vi "S2 Step Run For Program.vi"(8 "error in (no error)":errorcluster) -> (0 "error out":errorcluster)   [LabVIEW 2019]
uses:
  LineScan/LineScan.lvclass
  Ctrl/Station Action.ctl
  Ctrl/StationCmdSelect.ctl
  Ctrl/Auto Inspection Station Name2.ctl
  Ctrl/Auto Inspection Data Name.ctl
  Ctrl/MeasureDisplayTab.ctl
  Ctrl/Table Save.ctl
  Ctrl/S2 Station IO.ctl
  Global/Process Global.vi
  LLB/Commonly VI/Main Glb.vi
  LLB/Commonly VI.lvlib
panel:
  out "CurrentCmd 2":string
  out "retry次數 2":string[](array[string])
  out "Retry 2":i32
  in  "Table Control":string[][](table)=[["PCBA BARCODE", ""], ["硬體(Tool初始化)", ""], ["company(Tool初始化)", ""], ["耗電流 uA(電流表)", "T"], ["電池負載電壓", "T"], ["晶片ID(Tool FORMAT)", "F"], ["雷雕ID(TOOl scan、藍芽接收器)", "S"], ["Format(Tool FORMAT)", "F"], ["Programe(Tool Programe)", "P"]]
  out "Numeric":dbl
  out "subarray":string[](array[string])
  out "Program1 receive 2":string
  out "ToolStringOut_P1":string
  out "ToolStringOut_P1_2":string
  out "present":i32
  out "Retry":i32
  out "Act Step":i32
  out "retry次數":string[](array[string])
  out "CurrentCmd":string
  out "Station Out":T1=enum."ImformOut"
  out "LineScan out":refnum<class "LineScan.lvclass">
  in  "LineScan in":refnum<class "LineScan.lvclass">
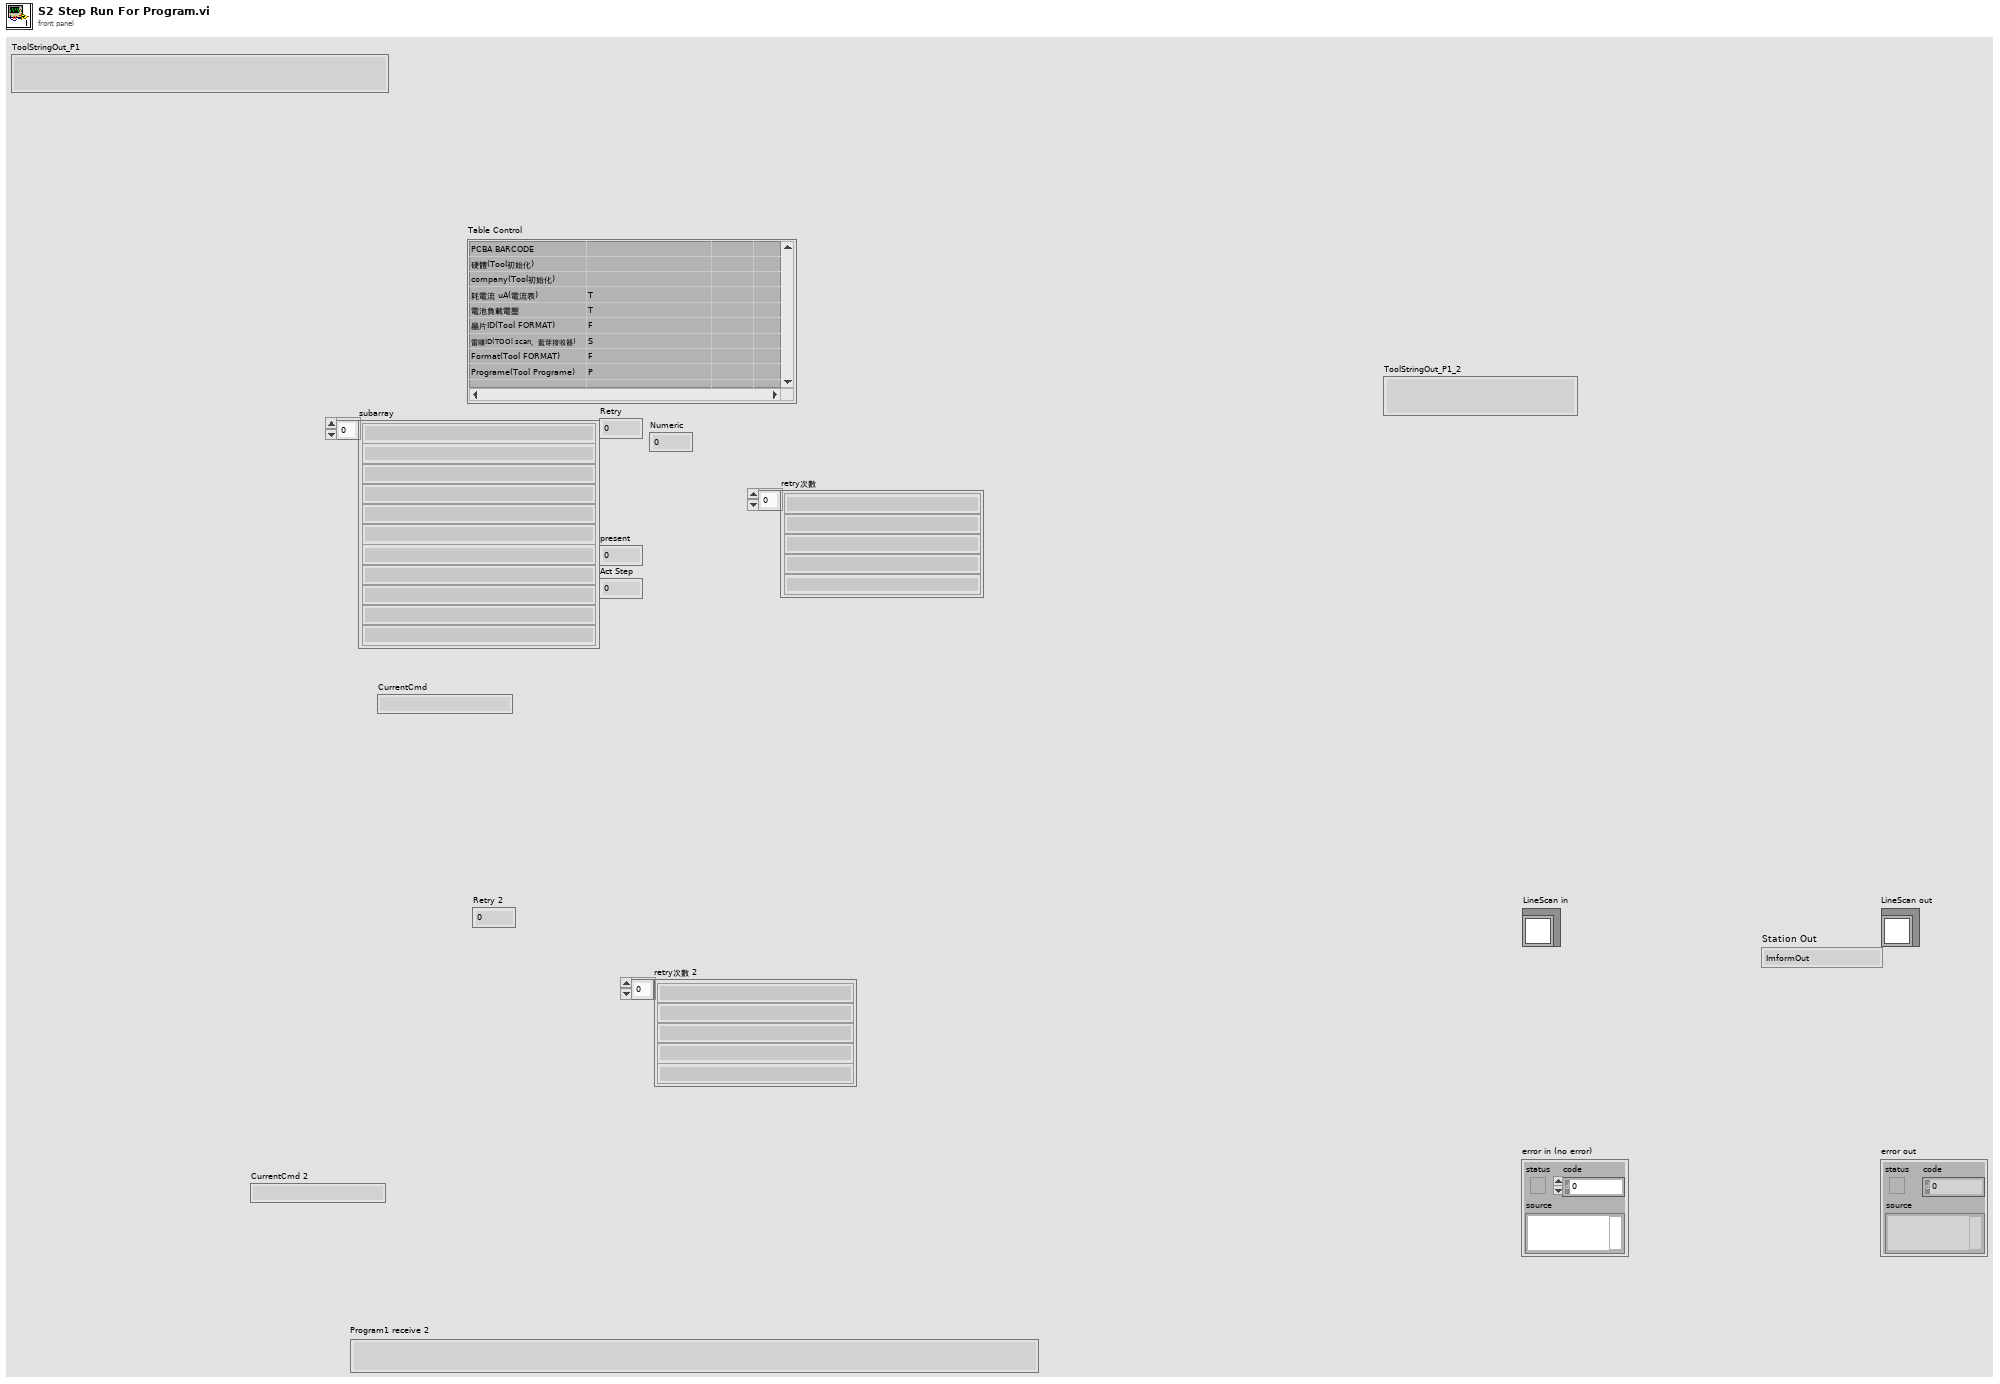
[diagram p1: front panel]
types:
  T1 = typedef "Station Action.ctl" = enum16{"Wait Item In", "Dectect Action", "ImformOut"}
  T2 = typedef "StationCmdSelect.ctl" = enum16{"Action", "Command", "Return", "DTime", "Retry"}
  T3 = typedef "Table Save.ctl" = enum16{"initial", "Add", "Write", "Replace", "Delete", "REad", "RedTable", "Load"}
  T4 = typedef "MeasureDisplayTab.ctl" = enum16{"Tray Barcode", "PCBA BARCODE", "硬體(Tool初始化)", "company(Tool初始化)", "耗電流 uA(電流表)", "電池負載電壓", "晶片ID(Tool FORMAT)", "雷雕ID(TOOl scan、藍芽接收器)", "Format(Tool FORMAT)", "Programe(Tool Programe)", "MAC(藍芽接收器)", "ID(藍芽接收器)", "KPA(藍芽接收器)", "溫度(藍芽接收器)", "SENSOR電池電壓(藍芽接收器)", "RSSI(藍芽接收器)", "SensorType_315(FSK scan)", "FSKsnVol_315(FSK scan)", "FSKscanl_315(FSK scan)", "P_315(FSK scan)", "T_315(FSK scan)", "SensorType_433(ASK scan)", "ASKsnVol_433(ASK scan)", "ASKscan_433(ASK scan)", "P_433(ASK scan)", "T_433(ASK scan)", "測高Data"}
  T5 = typedef "Auto Inspection Data Name.ctl" = enum16{"LocalRun", "ItemSN(TimeCode)", "CurrentAction", "Error", "Data", "OKNG", "電壓值", "電壓值判斷", "電流值", "電流值判斷", "Laser1 Data", "Laser2 Data", "Laser OKNG", "StationNO"}
  T6 = typedef "Auto Inspection Station Name2.ctl" = enum16{"S1Barcode", "S2Measure", "S3Measure", "S4Measure", "S5Measure", "S11_LaserCheck", "S8_Vision AI"}
  T7 = typedef "S2 Station IO.ctl" = enum16{"S2站PC動作中_20", "電流量測完成產品OK_21", "電流量測完成產品NG_22", "S2站Format 執行_23", "S2 Format OK_24", "S2 Format NG_25", "S2站燒入執行_26", "S2站燒入OK_27", "S2站燒入NG_28", "S2站動作完成_29", "S3 PC動作中_30", "S3 Format 此站執行_31", "S3 Format OK_32", "S3 Format NG_33", "S3 燒入程式 此站執行_34", "S3 燒入程式 OK_35", "S3 燒入程式 NG_36", "S3 備用_37", "S3 備用_38", "S3 動作完成_39", "S4 PC動作中_40", "S4 量測完成 產品正常_41", "S4 量測完成 產品NG_42", "S4 Format 此站執行_43", "S4 Format OK_44", "S4 Format NG_45", "S4 燒入 此站不執行_46", "S4 燒入程式 OK_47", "S4 燒入程式 NG_48", "S4 藍芽Scan OK_49", "S4 藍芽Scan NG_50", "S4 動作完成_51", "給PLC要量電流訊號", "給PLC要量電壓訊號"}
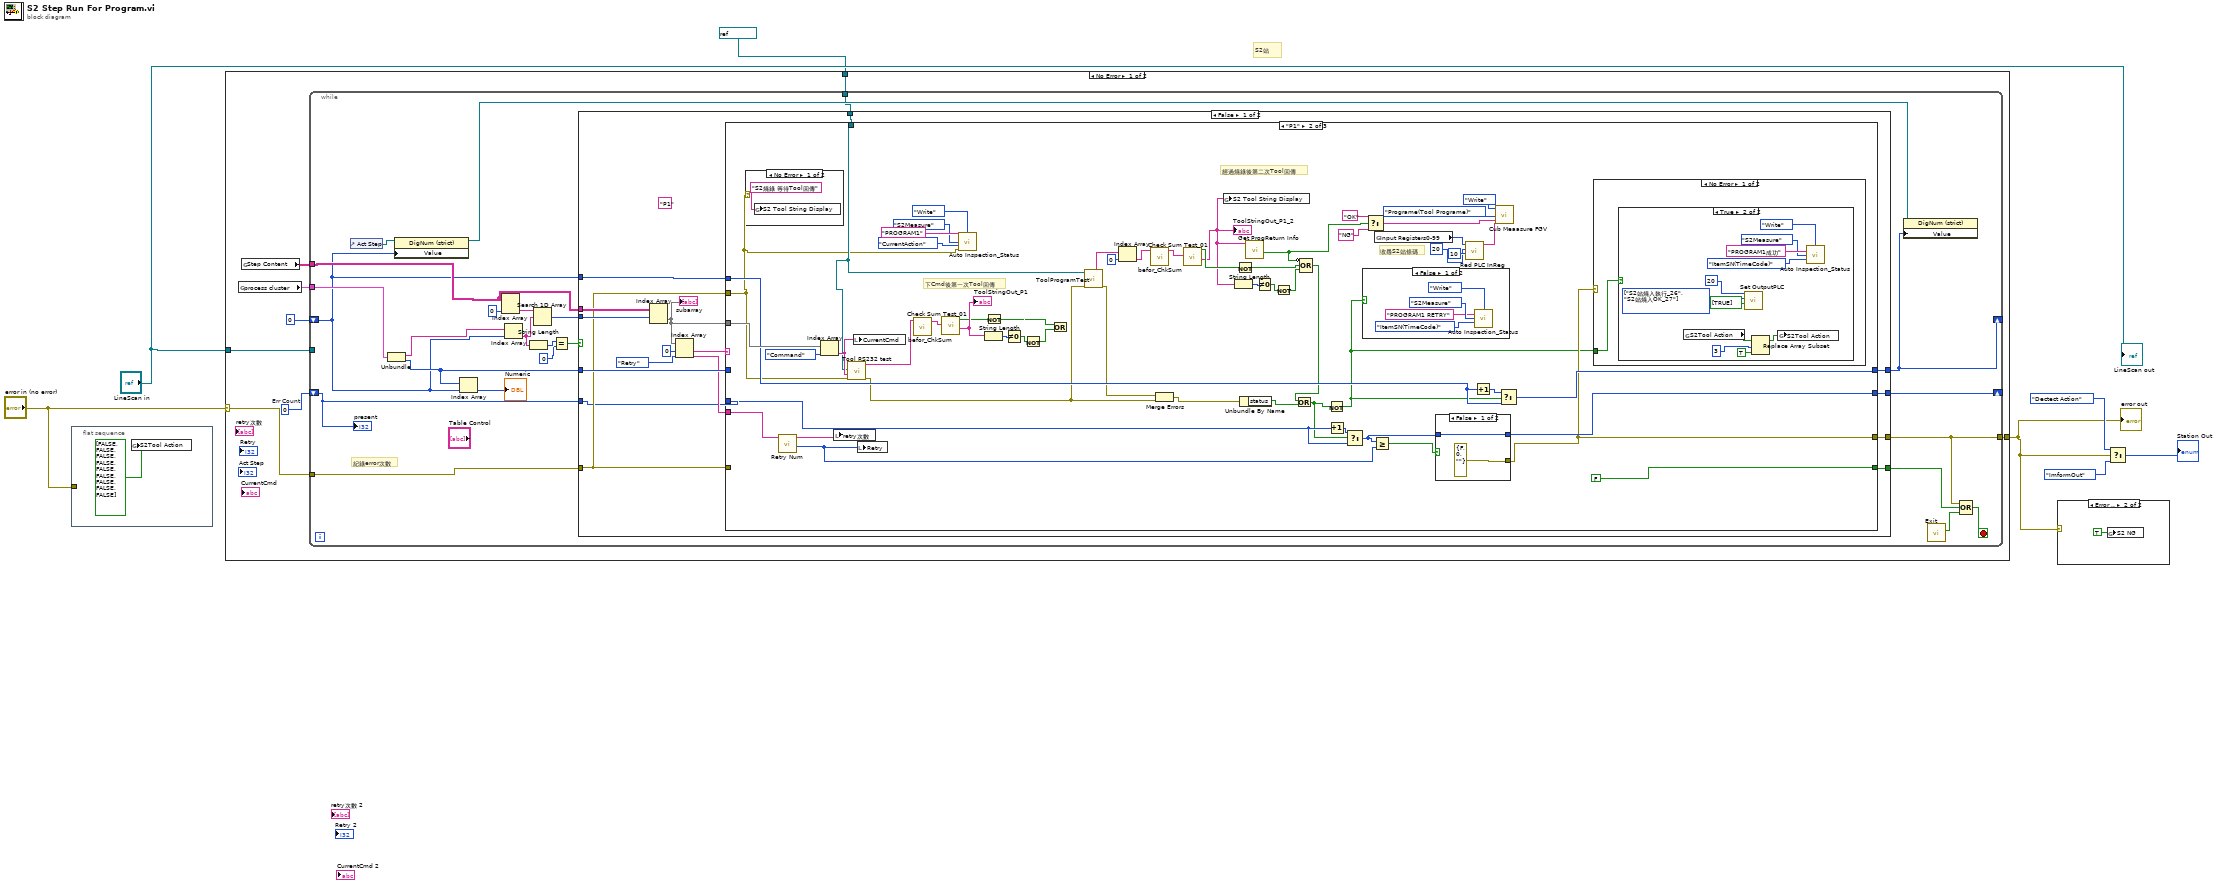
[diagram p0: block diagram]
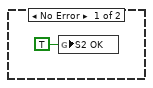
[diagram p2: hidden frame]
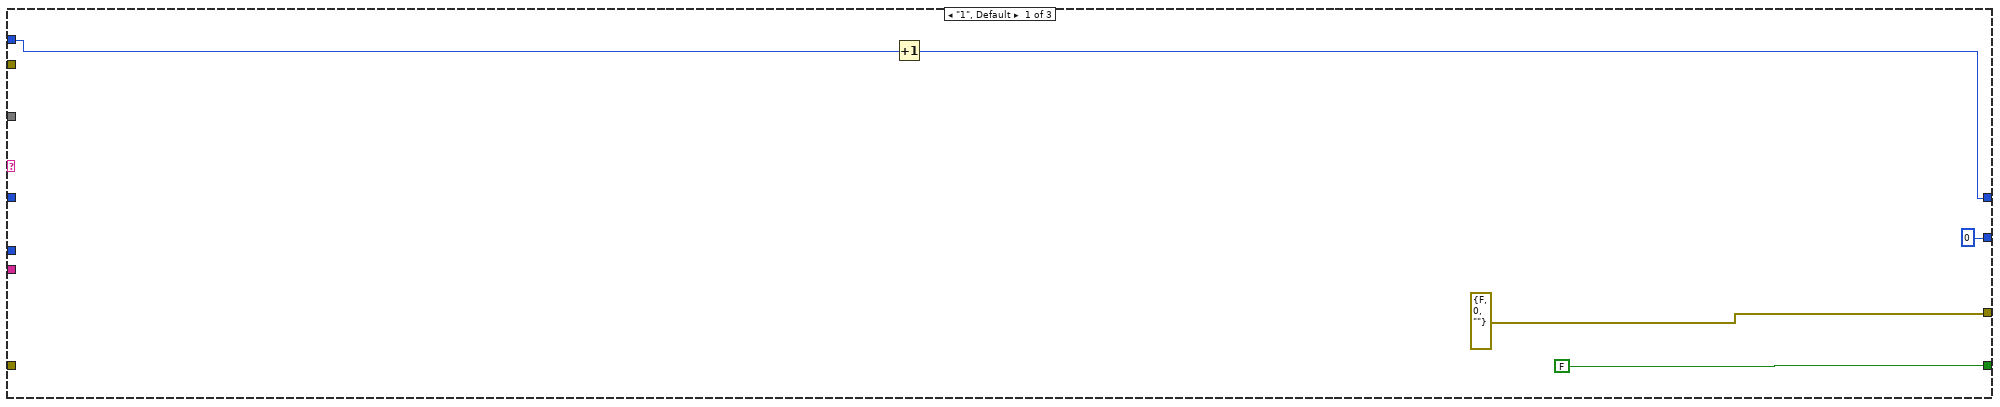
[diagram p3: hidden frame]
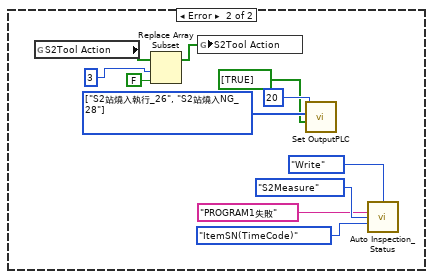
[diagram p7: hidden frame]
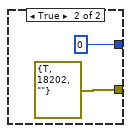
[diagram p8: hidden frame]
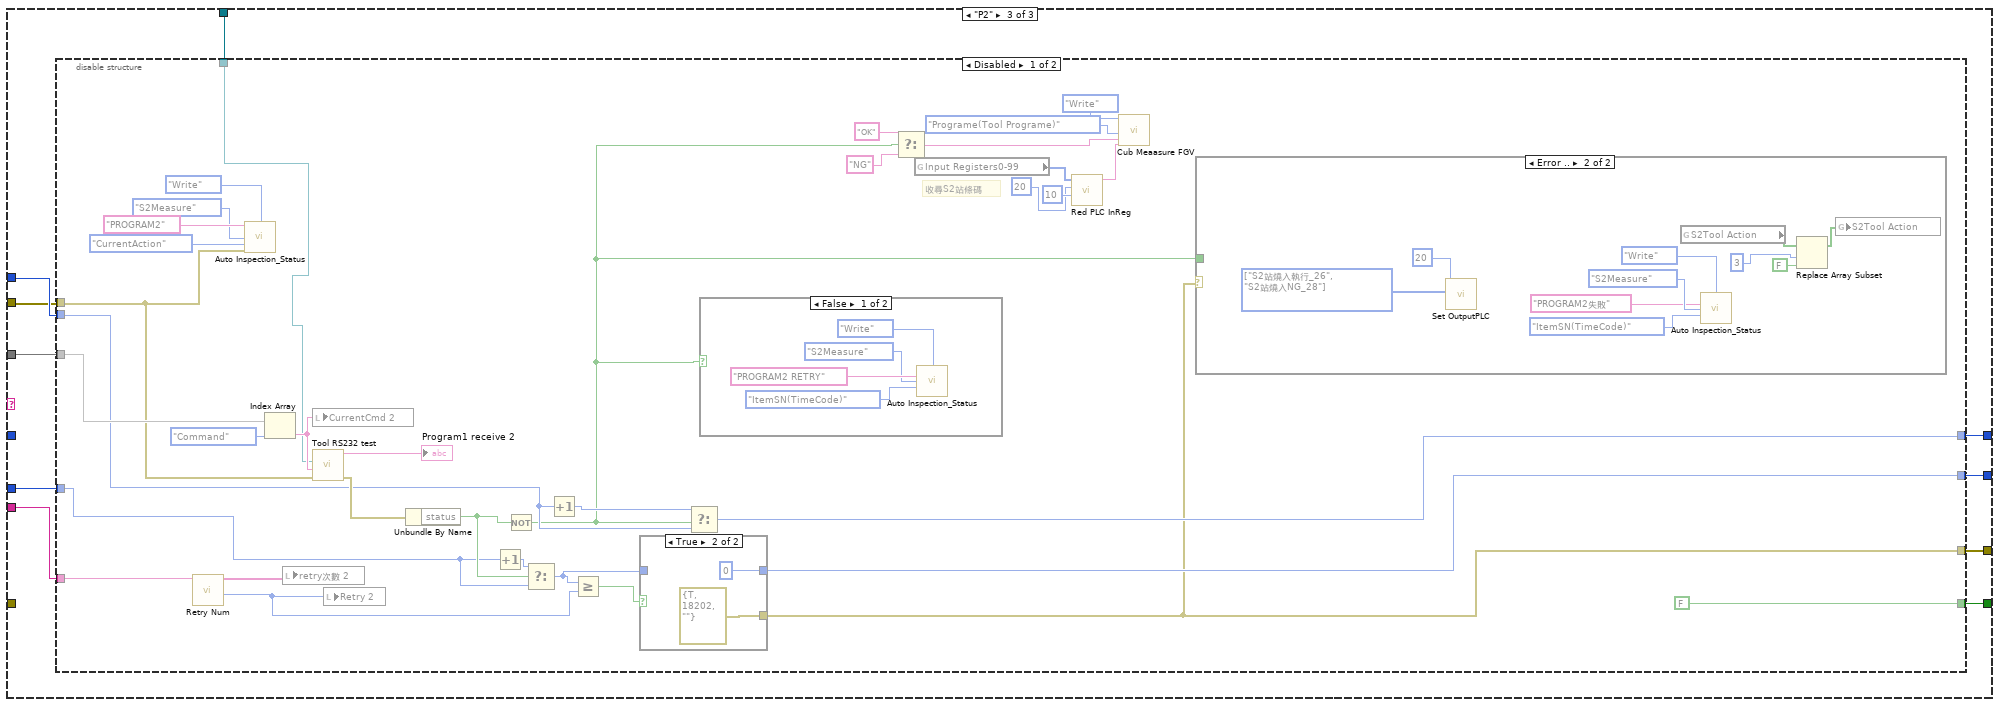
[diagram p9: hidden frame]
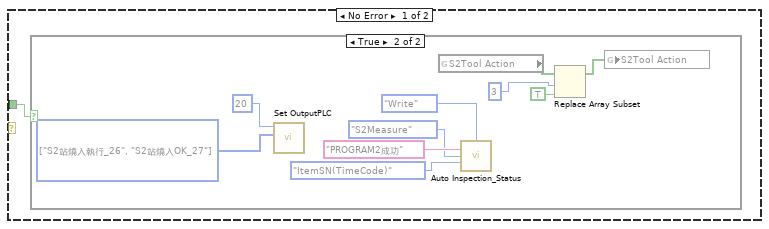
[diagram p11: hidden frame]
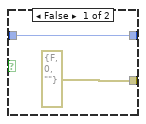
[diagram p13: hidden frame]
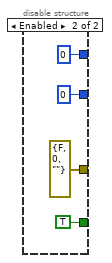
[diagram p14: hidden frame]
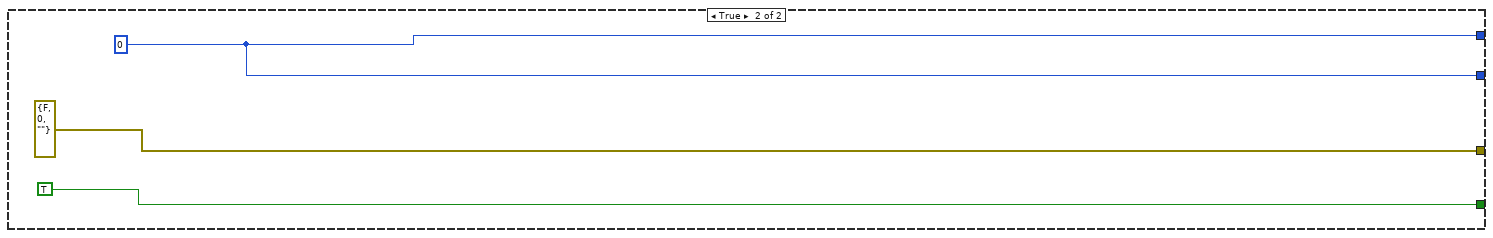
[diagram p15: hidden frame]
diagram:
  # "S2站"
  n1 = flat-sequence {
    tunnel: "error in (no error)" -> [_]
    frame #0 {
      n2 = global write "Process Global.vi" "S2Tool Action"(bool[] [FALSE, FALSE, FALSE, FALSE, FALSE, FALSE, FALSE, FALSE, FALSE] ("S2Tool Action")) -> ()
    }
  }
  n3 = case shown="No Error" "error in (no error)" {
    selector: "error in (no error)" -> [w10 w232]
    tunnel: [w16 w232] -> w2
    tunnel: "LineScan in" -> [w15 _]
    tunnel: refnum<visa-resource-name> "COM1" ("VISA resource name") -> [w9 _]
    frame No Error {
      w11 = 0  # Err Count
      n4 = global read "Process Global.vi" "process cluster"() -> (w13:cluster{string[], i32[]})
      n5 = global read "Process Global.vi" "Step Content"() -> (w14:string[][])
      n6 = while {
        tunnel: [w26] -> w16
        shift-right: [w22] -> _
        shift-left: 0 -> [w23]
        tunnel: w15 -> [_]
        shift-right: [w19] -> _
        shift-left: w11 -> [w25]
        tunnel: w14 -> [w37]
        tunnel: w13 -> [w36]
        tunnel: w10 -> [w20]
        tunnel: w9 -> [w18]
        stop <- w38 stop-if-true
        # "紀錄error次數"
        n7 = control-ref of="Act Step"() -> (w24:refnum<vi>)
        n8 = Unbundle(w36) -> (w39:string[], w40:i32[])
        n9 = property class="DigNum (strict)"(reference=w24, "Value"=w23) -> (reference out=w21:refnum<vi>)  [unwired: 1 in, 1 out]
        n10 = Index Array(array=w40, index=w23) -> (element=→"Numeric":i32)
        n11 = Index Array(array=w37, index (col)=0 ("disabled index (col)")) -> (element=w34:string[])  [unwired: 1 in]
        n12 = Index Array(array=w39, index=w23) -> (element=w30:string)
        n13 = String Length(string=w30) -> (length=w31:i32)
        n14 = Search 1D Array(1D array=w34, element=w30) -> (index of element=w33:i32)  [unwired: 1 in]
        n15 = Equal?(x=w31, y=0) -> (x = y?=w28:bool)
        n16 = case shown="False" w28 {
          tunnel: w40 -> [w56 _]
          tunnel: w37 -> [w55 _]
          tunnel: w33 -> [w54 _]
          tunnel: [w46 TRUE] -> w27
          tunnel: [w48 errorcluster {"status"=FALSE, "code"=0, "source"=""} ("error constant")] -> w26
          tunnel: w23 -> [w50 _]
          tunnel: [w49 w229] -> w22
          tunnel: w25 -> [w44 _]
          tunnel: w20 -> [w45 _]
          tunnel: [w43 w229] -> w19
          tunnel: w18 -> [w42 _]
          frame False {
            (unwired) "P1"
            n17 = Index Array(array=w55, index (row)=w54) -> (element=w51:string[])  [unwired: 1 in]
            "subarray" <- w51
            n18 = Index Array(array=w51, index #1=0 ("index"), index #2=StationCmdSelect."Retry") -> (element #1=w41:string, element #2=w52:string)
            n19 = case shown="\"P1\"" w41 {
              tunnel: w56 -> [_ _ _]
              tunnel: w52 -> [_ w108 w156]
              tunnel: w51 -> [_ w110 w159]
              tunnel: w50 -> [w61 w109 w158]
              tunnel: [w60 w107 w155] -> w49
              tunnel: [errorcluster {"status"=FALSE, "code"=0, "source"=""} ("error constant") w68 w152] -> w48
              tunnel: [FALSE FALSE w153] -> w46
              tunnel: w45 -> [_ _ _]
              tunnel: w45 -> [_ w66 w151]
              tunnel: w44 -> [_ w91 w157]
              tunnel: [0 ("Err Count") w92 w154] -> w43
              tunnel: w42 -> [_ w82 w160]
              frame "1", Default {
                n20 = Increment(x=w61) -> (x+1=w60:i32)
              }
              frame "P1" {
                # "經過燒錄後第二次Tool回傳"
                # "下Cmd後第一次Tool回傳"
                # "收尋S2站條碼"
                n21 = case shown="No Error" w66 {
                  frame No Error {
                    n22 = global write "Process Global.vi" "S2 Tool String Display"("S2燒錄 等待Tool回傳" ("S2 Tool String Display")) -> ()
                  }
                  frame Error {
                  }
                }
                n23 = call "Retry Num.vi"("String"=w108) -> ("Numeric"=w116:i32, "retry次數"=w113:string[])  [unwired: 9 in]
                n24 = Index Array(array=w110, index=StationCmdSelect."Command") -> (element=w112:string)
                n25 = local write "retry次數"(w113) -> ()
                n26 = call "Tool RS232 test.vi"("error in (no error)"=w66, "Cmd In"=w112, "VISA resource name"=w82) -> ("error out"=w63:errorcluster, "receive string"=w83:string)  [unwired: 7 in]
                n27 = local write "CurrentCmd"(w112) -> ()
                n28 = local write "Retry"(w116) -> ()
                n29 = call "befor_ChkSum.vi"("ToolString Input"=w83) -> ("Array"=w84:string[])  [unwired: 9 in, 1 out]
                n30 = call "Check Sum Test_01.vi"("Array"=w84) -> ("ToolStringOut_01"=w87:string, "x = y?"=w85:bool)  [unwired: 8 in, 1 out]
                "ToolStringOut_P1" <- w87
                n31 = call "Auto Inspection_Status.vi"("Action"=enum16{"Initial", "Write", "Read"}."Write", "DataIn"="PROGRAM1", "Station"=Auto_Inspection_Station_Name2."S2Measure", "Data"=Auto_Inspection_Data_Name."CurrentAction", "error in"=w66) -> ()  [unwired: 8 in, 3 out]
                n32 = String Length(string=w87) -> (length=w89:i32)
                n33 = Not(x=w85) -> (.not. x?=w86:bool)
                n34 = Not Equal To 0?(x=w89) -> (x != 0?=w90:bool)
                n35 = Not(x=w90) -> (.not. x?=w88:bool)
                n36 = Or(x=w86, y=w88) -> ()  [unwired: 1 out]
                n37 = call "ToolProgramTest.vi"("error in (no error)"=w63, "VISA resource name"=w82) -> ("error out"=w64:errorcluster, "Array"=w73:string[])  [unwired: 4 in, 4 out]
                n38 = Index Array(array=w73, index=0) -> (element=w80:string)
                n39 = call "befor_ChkSum.vi"("ToolString Input"=w80) -> ("Array"=w79:string[])  [unwired: 9 in, 1 out]
                n40 = Merge Errors(w64, w63) -> (w62:errorcluster)
                n41 = call "Check Sum Test_01.vi"("Array"=w79) -> ("ToolStringOut_01"=w67:string, "x = y?"=w76:bool)  [unwired: 8 in, 1 out]
                "ToolStringOut_P1_2" <- w67
                n42 = global write "Process Global.vi" "S2 Tool String Display"(w67) -> ()
                n43 = String Length(string=w67) -> (length=w77:i32)
                n44 = Not(x=w76) -> (.not. x?=w75:bool)
                n45 = Unbundle By Name(w62) -> ("status"=w71:bool)
                n46 = call "Get ProgReturn Info.vi"("String"=w67) -> ("Chk OK or Fail"=w72:bool)  [unwired: 8 in, 2 out]
                n47 = Not Equal To 0?(x=w77) -> (x != 0?=w78:bool)
                n48 = Not(x=w78) -> (.not. x?=w74:bool)
                n49 = Compound Arithmetic op=OR(invert w72, w75, w74) -> (w70:bool)
                n50 = Or(x=w70, y=w71) -> (x .or. y?=w69:bool)
                n51 = Not(x=w69) -> (.not. x?=w65:bool)
                n52 = Increment(x=w91) -> (x+1=w117:i32)
                n53 = Select(t=w117, s=w69, f=w91) -> (s? t:f=w114:i32)
                n54 = case shown="False" w65 {
                  frame False {
                    n55 = call "Auto Inspection_Status.vi"("Action"=enum16{"Initial", "Write", "Read"}."Write", "DataIn"="PROGRAM1 RETRY", "Station"=Auto_Inspection_Station_Name2."S2Measure", "Data"=Auto_Inspection_Data_Name."ItemSN(TimeCode)") -> ()  [unwired: 9 in, 3 out]
                  }
                  frame True {
                  }
                }
                n56 = Select(t="OK" ("DataIn"), s=w72, f="NG" ("DataIn")) -> (s? t:f=w101:string)
                n57 = Greater Or Equal?(x=w114, y=w116) -> (x >= y?=w115:bool)
                n58 = global read "Main Glb.vi" "Input Registers0-99"() -> (w94:u16[])
                n59 = case shown="False" w115 {
                  tunnel: [errorcluster {"status"=FALSE, "code"=0, "source"=""} ("error constant") errorcluster {"status"=TRUE, "code"=18202, "source"=""} ("error constant")] -> w68
                  tunnel: w114 -> [w147 _]
                  tunnel: [w147 0] -> w92
                  frame False {
                  }
                  frame True {
                  }
                }
                n60 = call "Red PLC InReg.vi"("length"=10, "index"=20, "Input Registers Arr"=w94) -> ("Rad In Reg"=w95:string)  [unwired: 7 in, 1 out]
                n61 = Increment(x=w109) -> (x+1=w118:i32)
                n62 = call "Cub Meaasure FGV.vi"("Action"=Table_Save."Write" ("Enum"), "Save Index"=MeasureDisplayTab."Programe(Tool Programe)", "DataIn"=w101, "SN"=w95) -> ()  [unwired: 8 in, 8 out]
                n63 = Select(t=w118, s=w65, f=w109) -> (s? t:f=w107:i32)
                n64 = case shown="No Error" w68 {
                  tunnel: w65 -> [w124 _]
                  frame No Error {
                    n65 = case shown="True" w124 {
                      frame False {
                      }
                      frame True {
                        w134 = T7[] [enum."S2站燒入執行_26", enum."S2站燒入OK_27"] items=["S2站PC動作中_20", "電流量測完成產品OK_21", "電流量測完成產品NG_22", "S2站Format 執行_23", "S2 Format OK_24", "S2 Format NG_25", "S2站燒入執行_26", "S2站燒入OK_27", "S2站燒入NG_28", "S2站動作完成_29", "S3 PC動作中_30", "S3 Format 此站執行_31", "S3 Format OK_32", "S3 Format NG_33", "S3 燒入程式 此站執行_34", "S3 燒入程式 OK_35", "S3 燒入程式 NG_36", "S3 備用_37", "S3 備用_38", "S3 動作完成_39", "S4 PC動作中_40", "S4 量測完成 產品正常_41", "S4 量測完成 產品NG_42", "S4 Format 此站執行_43", "S4 Format OK_44", "S4 Format NG_45", "S4 燒入 此站不執行_46", "S4 燒入程式 OK_47", "S4 燒入程式 NG_48", "S4 藍芽Scan OK_49", "S4 藍芽Scan NG_50", "S4 動作完成_51", "給PLC要量電流訊號", "給PLC要量電壓訊號"]
                        n66 = global read "Process Global.vi" "S2Tool Action"() -> (w129:bool[])
                        n67 = call "Set OutputPLC.vi"("Address In"=20, "Array 2"=w134, "Sat Coils"=bool[] [TRUE]) -> ()  [unwired: 7 in, 1 out]
                        n68 = Replace Array Subset(array=w129, new element=TRUE ("new element/subarray"), index=3) -> (w126:bool[])
                        n69 = global write "Process Global.vi" "S2Tool Action"(w126) -> ()
                        n70 = call "Auto Inspection_Status.vi"("Action"=enum16{"Initial", "Write", "Read"}."Write", "DataIn"="PROGRAM1成功", "Station"=Auto_Inspection_Station_Name2."S2Measure", "Data"=Auto_Inspection_Data_Name."ItemSN(TimeCode)") -> ()  [unwired: 9 in, 3 out]
                      }
                    }
                  }
                  frame Error {
                    w146 = T7[] [enum."S2站燒入執行_26", enum."S2站燒入NG_28"] items=["S2站PC動作中_20", "電流量測完成產品OK_21", "電流量測完成產品NG_22", "S2站Format 執行_23", "S2 Format OK_24", "S2 Format NG_25", "S2站燒入執行_26", "S2站燒入OK_27", "S2站燒入NG_28", "S2站動作完成_29", "S3 PC動作中_30", "S3 Format 此站執行_31", "S3 Format OK_32", "S3 Format NG_33", "S3 燒入程式 此站執行_34", "S3 燒入程式 OK_35", "S3 燒入程式 NG_36", "S3 備用_37", "S3 備用_38", "S3 動作完成_39", "S4 PC動作中_40", "S4 量測完成 產品正常_41", "S4 量測完成 產品NG_42", "S4 Format 此站執行_43", "S4 Format OK_44", "S4 Format NG_45", "S4 燒入 此站不執行_46", "S4 燒入程式 OK_47", "S4 燒入程式 NG_48", "S4 藍芽Scan OK_49", "S4 藍芽Scan NG_50", "S4 動作完成_51", "給PLC要量電流訊號", "給PLC要量電壓訊號"]
                    n71 = global read "Process Global.vi" "S2Tool Action"() -> (w140:bool[])
                    n72 = Replace Array Subset(array=w140, new element=FALSE ("new element/subarray"), index=3) -> (w137:bool[])
                    n73 = global write "Process Global.vi" "S2Tool Action"(w137) -> ()
                    n74 = call "Set OutputPLC.vi"("Address In"=20, "Array 2"=w146, "Sat Coils"=bool[] [TRUE]) -> ()  [unwired: 7 in, 1 out]
                    n75 = call "Auto Inspection_Status.vi"("Action"=enum16{"Initial", "Write", "Read"}."Write", "DataIn"="PROGRAM1失敗", "Station"=Auto_Inspection_Station_Name2."S2Measure", "Data"=Auto_Inspection_Data_Name."ItemSN(TimeCode)") -> ()  [unwired: 9 in, 3 out]
                  }
                }
              }
              frame "P2" {
                n76 = disable-structure shown="Disabled" {
                  disable-tunnel: w160 -> [w171 _]
                  disable-tunnel: w159 -> [w170 _]
                  disable-tunnel: w158 -> [w169 _]
                  disable-tunnel: w157 -> [w168 _]
                  disable-tunnel: w156 -> [w167 _]
                  disable-tunnel: [w166 0] -> w155
                  disable-tunnel: [w165 0 ("Err Count")] -> w154
                  disable-tunnel: [FALSE TRUE] -> w153
                  disable-tunnel: [w163 errorcluster {"status"=FALSE, "code"=0, "source"=""} ("error constant")] -> w152
                  disable-tunnel: w151 -> [w162 _]
                  frame Disabled {
                    # "收尋S2站條碼"
                    n77 = call "Retry Num.vi"("String"=w167) -> ("Numeric"=w188:i32, "retry次數"=w191:string[])  [unwired: 9 in]
                    n78 = call "Auto Inspection_Status.vi"("Action"=enum16{"Initial", "Write", "Read"}."Write", "DataIn"="PROGRAM2", "Station"=Auto_Inspection_Station_Name2."S2Measure", "Data"=Auto_Inspection_Data_Name."CurrentAction", "error in"=w162) -> ()  [unwired: 8 in, 3 out]
                    n79 = Index Array(array=w170, index=StationCmdSelect."Command") -> (element=w192:string)
                    n80 = local write "retry次數 2"(w191) -> ()
                    n81 = local write "CurrentCmd 2"(w192) -> ()
                    n82 = call "Tool RS232 test.vi"("error in (no error)"=w162, "Cmd In"=w192, "VISA resource name"=w171) -> ("error out"=w184:errorcluster, "receive string"=→"Program1 receive 2":string)  [unwired: 7 in]
                    n83 = local write "Retry 2"(w188) -> ()
                    n84 = Unbundle By Name(w184) -> ("status"=w186:bool)
                    n85 = Increment(x=w168) -> (x+1=w187:i32)
                    n86 = Not(x=w186) -> (.not. x?=w161:bool)
                    n87 = Select(t=w187, s=w186, f=w168) -> (s? t:f=w190:i32)
                    n88 = Increment(x=w169) -> (x+1=w185:i32)
                    n89 = Greater Or Equal?(x=w190, y=w188) -> (x >= y?=w189:bool)
                    n90 = case shown="True" w189 {
                      tunnel: [errorcluster {"status"=FALSE, "code"=0, "source"=""} ("error constant") errorcluster {"status"=TRUE, "code"=18202, "source"=""} ("error constant")] -> w163
                      tunnel: w190 -> [w221 _]
                      tunnel: [w221 0] -> w165
                      frame False {
                      }
                      frame True {
                      }
                    }
                    n91 = Select(t=w185, s=w161, f=w169) -> (s? t:f=w166:i32)
                    n92 = case shown="False" w161 {
                      frame False {
                        n93 = call "Auto Inspection_Status.vi"("Action"=enum16{"Initial", "Write", "Read"}."Write", "DataIn"="PROGRAM2 RETRY", "Station"=Auto_Inspection_Station_Name2."S2Measure", "Data"=Auto_Inspection_Data_Name."ItemSN(TimeCode)") -> ()  [unwired: 9 in, 3 out]
                      }
                      frame True {
                      }
                    }
                    n94 = Select(t="OK" ("DataIn"), s=w161, f="NG" ("DataIn")) -> (s? t:f=w193:string)
                    n95 = global read "Main Glb.vi" "Input Registers0-99"() -> (w195:u16[])
                    n96 = call "Red PLC InReg.vi"("length"=10, "index"=20, "Input Registers Arr"=w195) -> ("Rad In Reg"=w194:string)  [unwired: 7 in, 1 out]
                    n97 = call "Cub Meaasure FGV.vi"("Action"=Table_Save."Write" ("Enum"), "Save Index"=MeasureDisplayTab."Programe(Tool Programe)", "DataIn"=w193, "SN"=w194) -> ()  [unwired: 8 in, 8 out]
                    n98 = case shown="Error .." w163 {
                      tunnel: w161 -> [w200 _]
                      frame No Error {
                        n99 = case shown="True" w200 {
                          frame False {
                          }
                          frame True {
                            w209 = T7[] [enum."S2站燒入執行_26", enum."S2站燒入OK_27"] items=["S2站PC動作中_20", "電流量測完成產品OK_21", "電流量測完成產品NG_22", "S2站Format 執行_23", "S2 Format OK_24", "S2 Format NG_25", "S2站燒入執行_26", "S2站燒入OK_27", "S2站燒入NG_28", "S2站動作完成_29", "S3 PC動作中_30", "S3 Format 此站執行_31", "S3 Format OK_32", "S3 Format NG_33", "S3 燒入程式 此站執行_34", "S3 燒入程式 OK_35", "S3 燒入程式 NG_36", "S3 備用_37", "S3 備用_38", "S3 動作完成_39", "S4 PC動作中_40", "S4 量測完成 產品正常_41", "S4 量測完成 產品NG_42", "S4 Format 此站執行_43", "S4 Format OK_44", "S4 Format NG_45", "S4 燒入 此站不執行_46", "S4 燒入程式 OK_47", "S4 燒入程式 NG_48", "S4 藍芽Scan OK_49", "S4 藍芽Scan NG_50", "S4 動作完成_51", "給PLC要量電流訊號", "給PLC要量電壓訊號"]
                            n100 = call "Set OutputPLC.vi"("Address In"=20, "Array 2"=w209) -> ()  [unwired: 8 in, 1 out]
                            n101 = global read "Process Global.vi" "S2Tool Action"() -> (w204:bool[])
                            n102 = call "Auto Inspection_Status.vi"("Action"=enum16{"Initial", "Write", "Read"}."Write", "DataIn"="PROGRAM2成功", "Station"=Auto_Inspection_Station_Name2."S2Measure", "Data"=Auto_Inspection_Data_Name."ItemSN(TimeCode)") -> ()  [unwired: 9 in, 3 out]
                            n103 = Replace Array Subset(array=w204, new element=TRUE ("new element/subarray"), index=3) -> (w201:bool[])
                            n104 = global write "Process Global.vi" "S2Tool Action"(w201) -> ()
                          }
                        }
                      }
                      frame Error {
                        w220 = T7[] [enum."S2站燒入執行_26", enum."S2站燒入NG_28"] items=["S2站PC動作中_20", "電流量測完成產品OK_21", "電流量測完成產品NG_22", "S2站Format 執行_23", "S2 Format OK_24", "S2 Format NG_25", "S2站燒入執行_26", "S2站燒入OK_27", "S2站燒入NG_28", "S2站動作完成_29", "S3 PC動作中_30", "S3 Format 此站執行_31", "S3 Format OK_32", "S3 Format NG_33", "S3 燒入程式 此站執行_34", "S3 燒入程式 OK_35", "S3 燒入程式 NG_36", "S3 備用_37", "S3 備用_38", "S3 動作完成_39", "S4 PC動作中_40", "S4 量測完成 產品正常_41", "S4 量測完成 產品NG_42", "S4 Format 此站執行_43", "S4 Format OK_44", "S4 Format NG_45", "S4 燒入 此站不執行_46", "S4 燒入程式 OK_47", "S4 燒入程式 NG_48", "S4 藍芽Scan OK_49", "S4 藍芽Scan NG_50", "S4 動作完成_51", "給PLC要量電流訊號", "給PLC要量電壓訊號"]
                        n105 = call "Set OutputPLC.vi"("Address In"=20, "Array 2"=w220) -> ()  [unwired: 8 in, 1 out]
                        n106 = global read "Process Global.vi" "S2Tool Action"() -> (w214:bool[])
                        n107 = call "Auto Inspection_Status.vi"("Action"=enum16{"Initial", "Write", "Read"}."Write", "DataIn"="PROGRAM2失敗", "Station"=Auto_Inspection_Station_Name2."S2Measure", "Data"=Auto_Inspection_Data_Name."ItemSN(TimeCode)") -> ()  [unwired: 9 in, 3 out]
                        n108 = Replace Array Subset(array=w214, new element=FALSE ("new element/subarray"), index=3) -> (w211:bool[])
                        n109 = global write "Process Global.vi" "S2Tool Action"(w211) -> ()
                      }
                    }
                  }
                  frame Enabled {
                  }
                }
              }
            }
          }
          frame True {
            w229 = 0
          }
        }
        n110 = property class="DigNum (strict)"(reference=w21, "Value"=w22) -> ()  [unwired: 1 in, 2 out]
        n111 = call "Exit.vi"() -> ("ExitOut"=w17:bool)  [unwired: 11 in]
        n112 = Compound Arithmetic op=OR(w26, w27, w17) -> (w38:bool)
        "present" <- w25
      }
    }
    frame Error {
    }
  }
  "error out" <- w2
  n113 = case shown="Error .." w2 {
    frame No Error {
      n114 = global write "Process Global.vi" "S2 OK"(TRUE ("S2 OK")) -> ()
    }
    frame Error {
      n115 = global write "Process Global.vi" "S2 NG"(TRUE ("S2 NG")) -> ()
    }
  }
  n116 = Select(t=Station_Action."Dectect Action" ("Station Out"), s=w2, f=Station_Action."ImformOut" ("Station Out")) -> (s? t:f=→"Station Out":T1)
  "LineScan out" <- "LineScan in"
